vi "VISA Read with Timeout.vi"(5 "error in (no error)":errorcluster, 6 "Timeout Limit":u32=5, 7 "Bytes to Read":u32=10, 8 "serial in":refnum<visa-resource-name>) -> (0 "error out":errorcluster, 1 "Error Out":bool, 2 "Timeout":bool, 3 "Serial Read":string, 4 "duplicate serial in":refnum<visa-resource-name>)   [LabVIEW 2019]
doc: "\"VISA Read with Timeout.VI\" deriva da \"Serial Read with Timeout.VI\" con le modifiche necessarie per il funzionamento con VISA.\nAutore: BOSCOLO ANDREA\nData: 21/7/2011"
panel:
  # "PC:  0 = COM1, 1= COM2,...\nMac:  0 = Modem, 1 = Printer\nSun: 0 = ttya, 1 = ttyb,..."
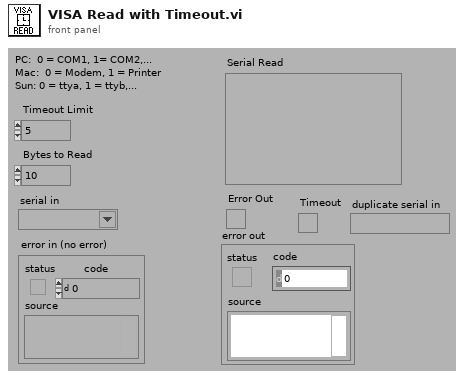
[diagram p1: front panel]
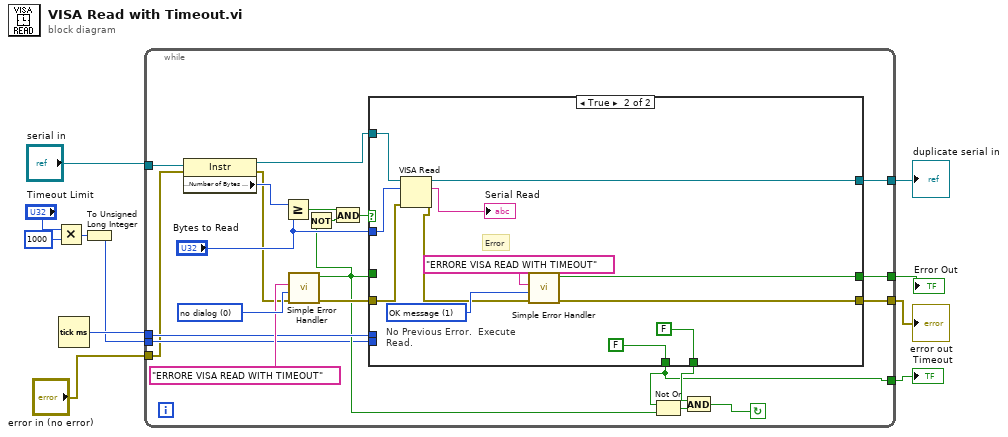
[diagram p0: block diagram]
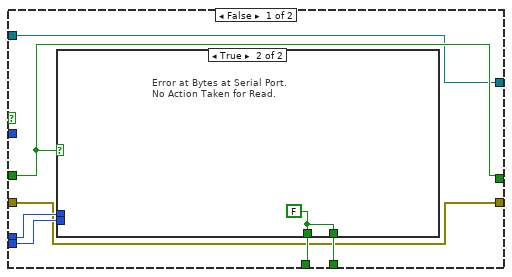
[diagram p2: hidden frame]
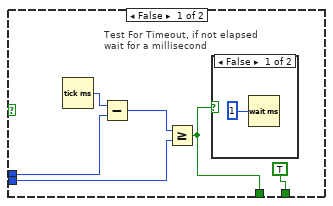
[diagram p3: hidden frame]
diagram:
  n1 = Multiply(x="Timeout Limit", y=u32 1000) -> (x*y=w6:u32)
  n2 = Tick Count (ms)() -> (millisecond timer value=w11:u32)
  n3 = To Unsigned Long Integer(number=w6) -> (unsigned 32bit integer=w5:u32)
  n4 = while {
    tunnel: w5 -> [w19]
    tunnel: [w21] -> w9
    tunnel: [w32] -> w10
    tunnel: w11 -> [w22]
    tunnel: "serial in" -> [w18]
    tunnel: "error in (no error)" -> [w13]
    tunnel: [w15] -> w1
    tunnel: [w14] -> w2
    stop <- w23 continue-if-true
    w27 = 0 items=["no dialog", "OK message", "continue or stop message"] ("type of dialog (OK msg:1)")
    n5 = property class="Instr"(reference=w18, error in=w13) -> (reference out=w16:refnum<visa-resource-name>, error out=w12:errorcluster, "Serial Settings:Number of Bytes at Serial Port"=w17:u32)
    n6 = Greater Or Equal?(x=w17, y="Bytes to Read") -> (x >= y?=w30:bool)
    n7 = call <vilib>:"Simple Error Handler.vi"("error source (\" \")"="ERRORE VISA READ WITH TIMEOUT", "type of dialog (OK msg:1)"=w27, "error in (no error)"=w12) -> ("error?"=w20:bool, "error out"=w28:errorcluster)  [unwired: 2 in, 3 out]
    n8 = Not(x=w20) -> (.not. x?=w29:bool)
    n9 = And(x=w30, y=w29) -> (x .and. y?=w31:bool)
    n10 = case shown="True" w31 {
      tunnel: "Bytes to Read" -> [_ w54]
      tunnel: [w38 w60] -> w32
      tunnel: w20 -> [w38 _]
      tunnel: w28 -> [w34 w52]
      tunnel: [w40 FALSE] -> w24
      tunnel: w22 -> [w39 _]
      tunnel: [w37 FALSE] -> w21
      tunnel: w19 -> [w36 _]
      tunnel: w16 -> [w35 w55]
      tunnel: [w34 w50] -> w15
      tunnel: [w35 w49] -> w14
      frame False {
        n11 = case shown="True" w38 {
          tunnel: [TRUE w48] -> w40
          tunnel: w39 -> [w44 _]
          tunnel: [w43 w48] -> w37
          tunnel: w36 -> [w41 _]
          frame False {
            # "Test For Timeout, if not elapsed\nwait for a millisecond"
            n12 = Tick Count (ms)() -> (millisecond timer value=w45:u32)
            n13 = Subtract(x=w45, y=w44) -> (x-y=w42:u32)
            n14 = Greater Or Equal?(x=w42, y=w41) -> (x >= y?=w43:bool)
            n15 = case shown="False" w43 {
              frame False {
                n16 = Wait (ms)(milliseconds to wait=u32 1 ("f")) -> ()  [unwired: 1 out]
              }
              frame True {
              }
            }
          }
          frame True {
            w48 = FALSE
            # "Error at Bytes at Serial Port.\nNo Action Taken for Read."
          }
        }
      }
      frame True {
        w56 = 1 items=["no dialog", "OK message", "continue or stop message"] ("type of dialog (OK msg:1)")
        # "No Previous Error.  Execute\nRead."
        # "Error"
        n17 = VISA Read(VISA resource name=w55, byte count=w54, error in (no error)=w52) -> (VISA resource name out=w49:refnum<visa-resource-name>, read buffer=→"Serial Read":string, error out=w51:errorcluster)  [unwired: 1 out]
        n18 = call <vilib>:"Simple Error Handler.vi"("error source (\" \")"="ERRORE VISA READ WITH TIMEOUT", "type of dialog (OK msg:1)"=w56, "error in (no error)"=w51) -> ("error?"=w60:bool, "error out"=w50:errorcluster)  [unwired: 2 in, 3 out]
      }
    }
    n19 = Not Or(1:w20, 2:w21) -> (0:w25:bool)
    n20 = And(x=w24, y=w25) -> (x .and. y?=w23:bool)
  }
  "Error Out" <- w10
  "Timeout" <- w9
  "duplicate serial in" <- w2
  "error out" <- w1
